vi "SubPanel_test.vi"() -> ()   [LabVIEW 2019]
panel:
  in  "stop":bool
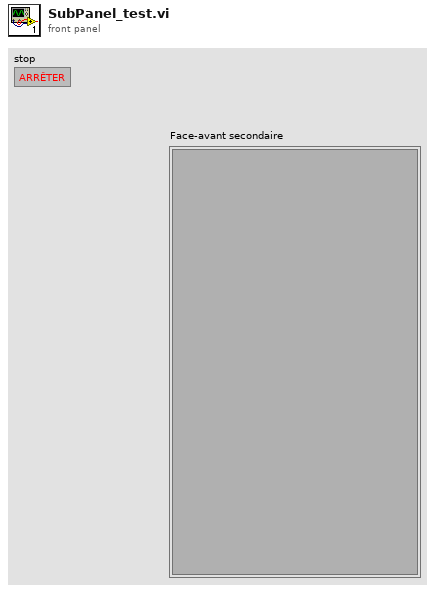
[diagram p1: front panel]
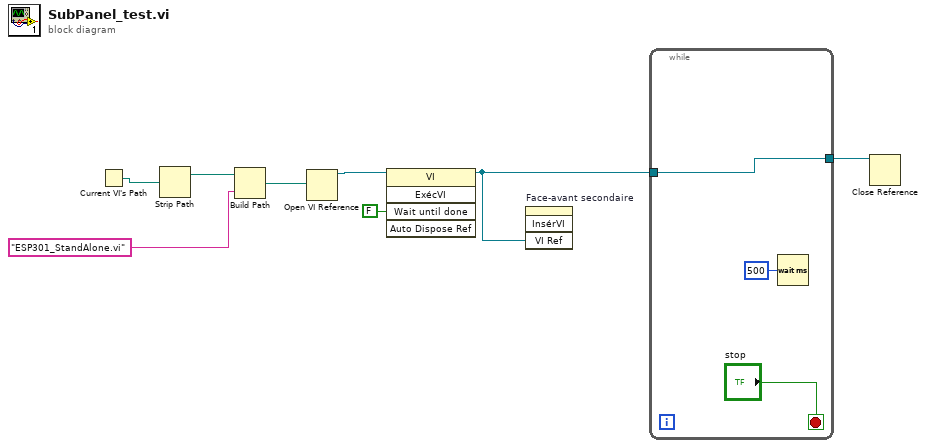
[diagram p0: block diagram]
diagram:
  n1 = Current VI's Path() -> (path=w5:path)
  n2 = Strip Path(path=w5) -> (stripped path=w6:path)  [unwired: 1 out]
  n3 = Build Path(base path=w6, name or relative path="ESP301_StandAlone.vi" ("nom ou chemin relatif")) -> (appended path=w7:path)
  n4 = Open VI Reference(vi path=w7) -> (vi reference=w8:refnum<vi>)  [unwired: 5 in, 1 out]
  n5 = invoke class="VI" method="ExécVI"(reference=w8, "Wait until done"=FALSE ("Attendre la fin")) -> (reference out=w2:refnum<vi>)  [unwired: 3 in, 4 out]
  n6 = invoke on="Face-avant secondaire" class="FAsec" method="InsérVI"("VI Ref"=w2) -> ()  [unwired: 3 in, 4 out]
  n7 = while {
    tunnel: [w10] -> w3
    tunnel: w2 -> [w10]
    stop <- "stop" stop-if-true
    n8 = Wait (ms)(milliseconds to wait=u32 500 ("attente (ms)")) -> ()  [unwired: 1 out]
  }
  n9 = Close Reference(reference=w3) -> ()  [unwired: 1 in, 1 out]
